vi "试剂余量设置.vi"(8 "Error in":errorcluster caption="Error in (no error)", 10 "试剂余量":T1, 11 "MB session in":refnum<class "MB_Master.lvclass">) -> (0 "error out":errorcluster, 3 "MB session out":refnum<class "MB_Master.lvclass">)   [LabVIEW 2016, in "斯坦道CODMn新电路板.lvlib"]
uses:
  <vilib>/Plasmionique/MB Master/MB_Master/MB_Master.lvclass
  <vilib>/Plasmionique/MB Master/MB Master.lvlib
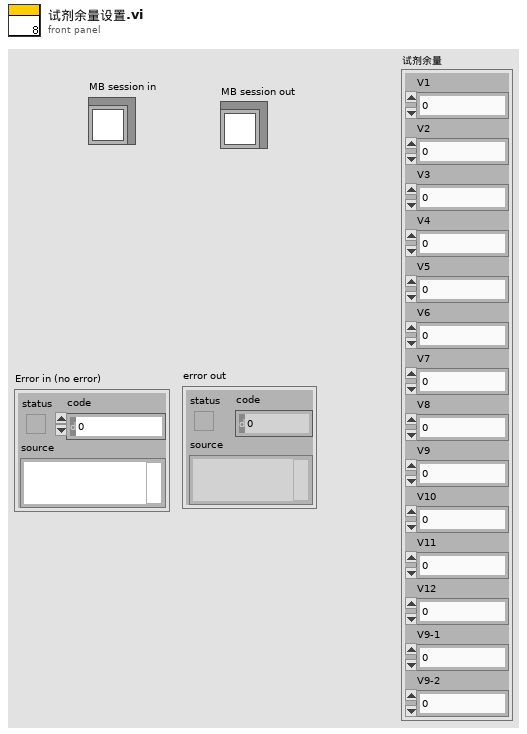
[diagram p1: front panel]
types:
  T1 = cluster{"V1":sgl, "V2":sgl, "V3":sgl, "V4":sgl, "V5":sgl, "V6":sgl, "V7":sgl, "V8":sgl, "V9":sgl, "V10":sgl, "V11":sgl, "V12":sgl, "V9-1":sgl, "V9-2":sgl}
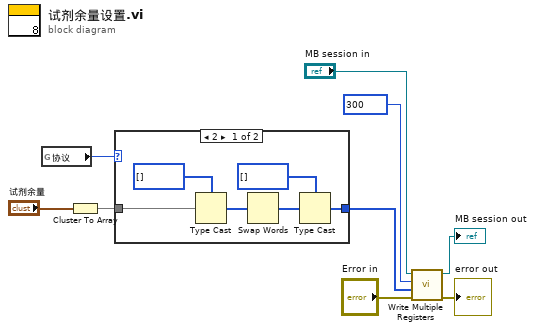
[diagram p0: block diagram]
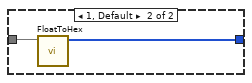
[diagram p2: hidden frame]
diagram:
  n1 = global read "CODMn断电保存全局变量.vi" "协议"() -> (w3:u16)
  n2 = Cluster To Array(cluster="试剂余量") -> (array=w2:sgl[])
  n3 = case shown="2" w3 {
    tunnel: [w10 w17] -> w1
    tunnel: w2 -> [w14 w16]
    frame 2 {
      n4 = Type Cast(type=u32[] [], x=w14) -> (*(type *) &x=w13:u32[])
      n5 = Swap Words(1:w13) -> (0:w11:u32[])
      n6 = Type Cast(type=u16[] [], x=w11) -> (*(type *) &x=w10:u16[])
    }
    frame 1, Default {
      n7 = call "FloatToHex.vi"("浮点数"=w16) -> ("DCBA整形输出"=w17:u16[])  [unwired: 10 in]
    }
  }
  n8 = call <vilib>:"Write Multiple Registers.vi"("error in (no error)"="Error in", "values"=w1, "starting address"=u16 300, "MB session in"="MB session in") -> ("error out"=→"error out":errorcluster, "MB session out"=→"MB session out":refnum<class "MB_Master.lvclass">)  [unwired: 6 in]
